vi "624ArcadeDriveHelper.vi"(9 "Y Power 2":dbl format="%#_13g", 10 "Y Power":dbl, 11 "Turn Power":dbl) -> (2 "Left":dbl, 3 "Right":dbl)   [LabVIEW 2015]
uses:
  Common Code/Drivetrain Modes.ctl
  Robot Code/Robot Global Data.vi
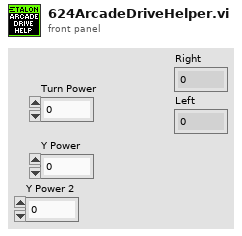
[diagram p1: front panel]
types:
  T1 = typedef "Drivetrain Modes.ctl" = enum16{"Tank", "Climb", "Manual", "Ball Vision Targeting", "Goal Vision Targeting", "PID Distance Drive", "Hybrid"}
  T2 = typedef "Drivetrain Commands.ctl" = cluster{"Y Power":dbl, "Turn Power":dbl, "1st Gear?":bool, "Modes":T1, "Heading Target":dbl, "X Max Speed":dbl, "Y Max Speed":dbl, "X Min Speed":dbl, "Y Min Speed":dbl, "Y Target":dbl, "Max Accel":dbl, "Max Velocity":dbl, "Y Power 2":dbl}
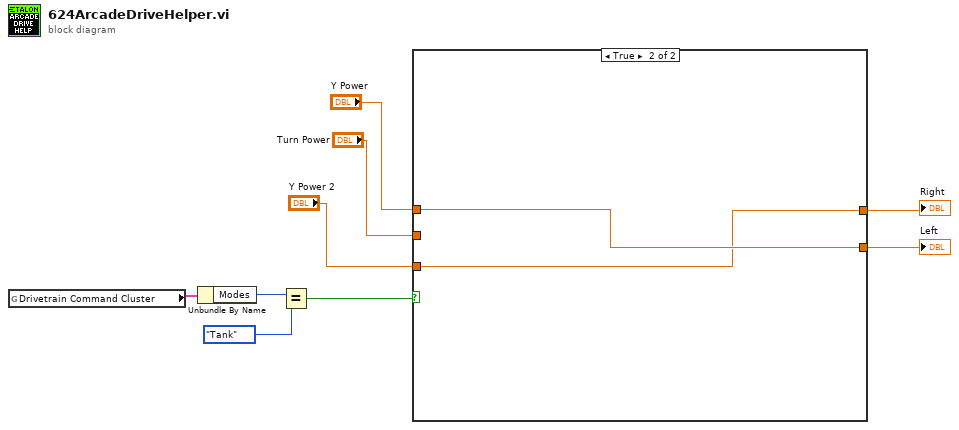
[diagram p0: block diagram]
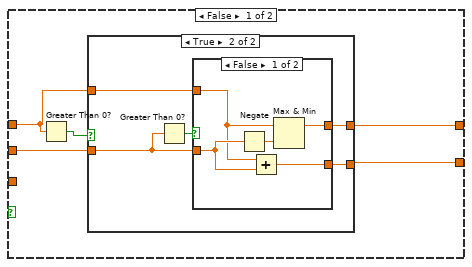
[diagram p2: hidden frame]
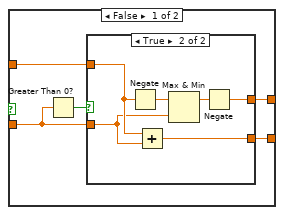
[diagram p3: hidden frame]
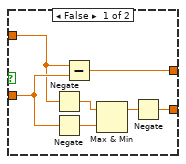
[diagram p4: hidden frame]
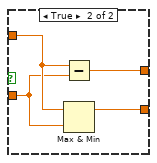
[diagram p5: hidden frame]
diagram:
  n1 = global read "Robot Global Data.vi" "Drivetrain Command Cluster"() -> (w6:T2)
  n2 = Unbundle By Name(w6) -> ("Modes"=w5:T1)
  n3 = Equal?(x=w5, y=Drivetrain_Modes."Tank") -> (x = y?=w7:bool)
  n4 = case shown="True" w7 {
    tunnel: "Turn Power" -> [w14 _]
    tunnel: "Y Power" -> [w13 w48]
    tunnel: "Y Power 2" -> [_ w47]
    tunnel: [w11 w47] -> w2
    tunnel: [w10 w48] -> w1
    frame False {
      n5 = Greater Than 0?(x=w13) -> (x > 0?=w12:bool)
      n6 = case shown="True" w12 {
        tunnel: w14 -> [w18 w36]
        tunnel: w13 -> [w17 w35]
        tunnel: [w16 w34] -> w11
        tunnel: [w15 w33] -> w10
        frame False {
          n7 = Greater Than 0?(x=w18) -> (x > 0?=w19:bool)
          n8 = case shown="True" w19 {
            tunnel: w18 -> [w26 w28]
            tunnel: w17 -> [w24 w29]
            tunnel: [w20 w30] -> w16
            tunnel: [w21 w27] -> w15
            frame False {
              n9 = Negate(x=w24) -> (-x=w25:dbl)
              n10 = Negate(x=w26) -> (-x=w23:dbl)
              n11 = Subtract(x=w24, y=w26) -> (x-y=w20:dbl)
              n12 = Max & Min(x=w25, y=w23) -> (max(x,y)=w22:dbl)  [unwired: 1 out]
              n13 = Negate(x=w22) -> (-x=w21:dbl)
            }
            frame True {
              n14 = Negate(x=w29) -> (-x=w32:dbl)
              n15 = Add(x=w29, y=w28) -> (x+y=w27:dbl)
              n16 = Max & Min(x=w32, y=w28) -> (max(x,y)=w31:dbl)  [unwired: 1 out]
              n17 = Negate(x=w31) -> (-x=w30:dbl)
            }
          }
        }
        frame True {
          n18 = Greater Than 0?(x=w36) -> (x > 0?=w37:bool)
          n19 = case shown="False" w37 {
            tunnel: w36 -> [w42 w44]
            tunnel: w35 -> [w39 w45]
            tunnel: [w40 w43] -> w34
            tunnel: [w38 w46] -> w33
            frame False {
              n20 = Negate(x=w42) -> (-x=w41:dbl)
              n21 = Add(x=w39, y=w42) -> (x+y=w38:dbl)
              n22 = Max & Min(x=w39, y=w41) -> (max(x,y)=w40:dbl)  [unwired: 1 out]
            }
            frame True {
              n23 = Subtract(x=w45, y=w44) -> (x-y=w43:dbl)
              n24 = Max & Min(x=w45, y=w44) -> (max(x,y)=w46:dbl)  [unwired: 1 out]
            }
          }
        }
      }
    }
    frame True {
    }
  }
  "Right" <- w2
  "Left" <- w1
